vi "ZXing.vi"(3 "二维码保存路径":string, 9 "height":i32, 10 "width":i32=100, 11 "contents":string) -> (2 "引用输出":refnum<k24>)   [LabVIEW 2020]
uses:
  ZXing/zxing.dll
  System.Drawing
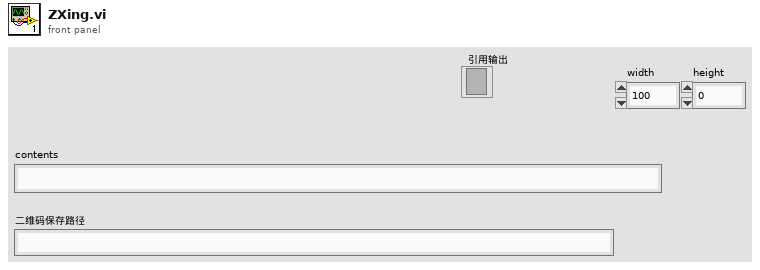
[diagram p1: front panel]
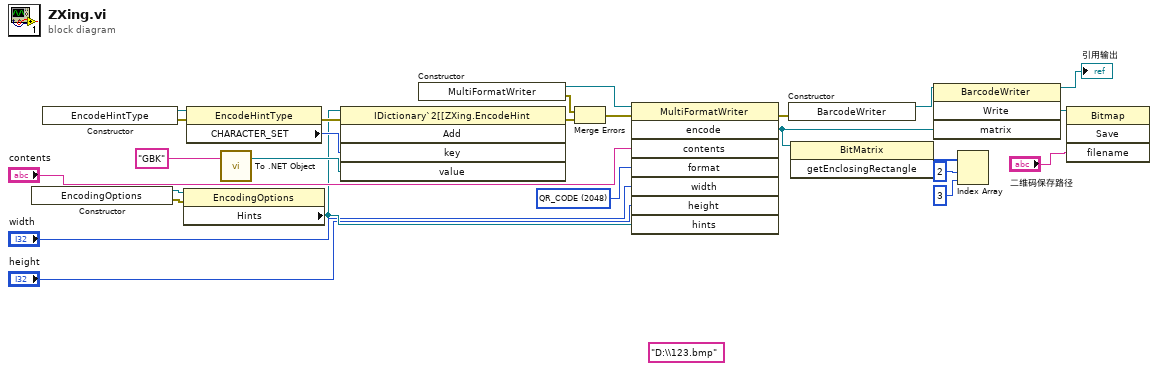
[diagram p0: block diagram]
diagram:
  w14 = 2048 items=["AZTEC"=1, "CODABAR"=2, "CODE_39"=4, "CODE_93"=8, "CODE_128"=16, "DATA_MATRIX"=32, "EAN_8"=64, "EAN_13"=128, "ITF"=256, "MAXICODE"=512, "PDF_417"=1024, "QR_CODE"=2048, "RSS_14"=4096, "RSS_EXPANDED"=8192, "UPC_A"=16384, "UPC_E"=32768, "All_1D"=61918, "UPC_EAN_EXTENSION"=65536, "MSI"=131072, "PLESSEY"=262144, "IMB"=524288] ("format")
  (unwired) "D:\\123.bmp" ("filename")
  n1 = constructor class="EncodingOptions"() -> (reference out=w18:refnum<k24>, error out=w19:errorcluster)  [unwired: 3 in, 1 out]
  n2 = constructor class="EncodeHintType"() -> (reference out=w20:refnum<k24>, error out=w23:errorcluster)  [unwired: 3 in, 1 out]
  n3 = property class="EncodingOptions"(reference=w18, error in=w19) -> ("Hints"=w15:refnum<k24>)  [unwired: 2 out]
  n4 = property class="EncodeHintType"(reference=w20, error in=w23) -> (error out=w24:errorcluster, "CHARACTER_SET"=w21:i32)  [unwired: 1 out]
  n5 = call <vilib>:"To .NET Object.vi"("anything"="GBK") -> (".NET object"=w22:refnum<k24>)  [unwired: 1 in, 1 out]
  n6 = invoke class="IDictionary`2[[ZXing.EncodeHint" method="Add"(reference=w15, error in=w24, "key"=w21, "value"=w22) -> (error out=w16:errorcluster)  [unwired: 1 in, 4 out]
  n7 = constructor class="MultiFormatWriter"() -> (reference out=w10:refnum<k24>, error out=w12:errorcluster)  [unwired: 3 in, 1 out]
  n8 = Merge Errors(w12, w16) -> (w11:errorcluster)
  n9 = invoke class="MultiFormatWriter" method="encode"(reference=w10, error in=w11, "contents"="contents", "format"=w14, "width"="width", "height"="height", "hints"=w15) -> (error out=w8:errorcluster, "encode"=w7:refnum<k24>)  [unwired: 1 in, 6 out]
  n10 = constructor class="BarcodeWriter"(error in=w8) -> (reference out=w9:refnum<k24>)  [unwired: 2 in, 2 out]
  n11 = invoke class="BitMatrix" method="getEnclosingRectangle"(reference=w7) -> ("getEnclosingRectangle"=w6:i32[])  [unwired: 2 in, 2 out]
  n12 = invoke class="BarcodeWriter" method="Write"(reference=w9, "matrix"=w7) -> (reference out=→"引用输出":refnum<k24>, "Write"=w26:refnum<k24>)  [unwired: 2 in, 2 out]
  n13 = Index Array(array=w6, index #1=2 ("索引"), index #2=3 ("索引")) -> ()  [unwired: 2 out]
  n14 = invoke class="Bitmap" method="Save"(reference=w26, "filename"="二维码保存路径") -> ()  [unwired: 2 in, 4 out]
